vi "Untitled 11 (SubVI).vi"(6 "Number of SPI Buses in":i32, 7 "Device Info":T1, 8 "error in (no error)":errorcluster, 9 "VI to which to Add Engines and IO Nodes":path, 10 "LabVIEW Project to Script":path, 11 "Curent Bus Path":path) -> (0 "error out":errorcluster, 3 "Number of SPI Buses out":i32)   [LabVIEW 2014, in "SPI Engine Scripting.lvlib"]
uses:
  SPI Engine Scripting.lvlib
  State Machine/Controls/Device Information.ctl
  State Machine/Controls/Pin Information.ctl
  State Machine/Controls/Bus Information.ctl
  <vilib>/LabVIEW Icon API/API_Text.ctl
  <vilib>/LabVIEW Icon API/LabVIEW Icon API.lvlib
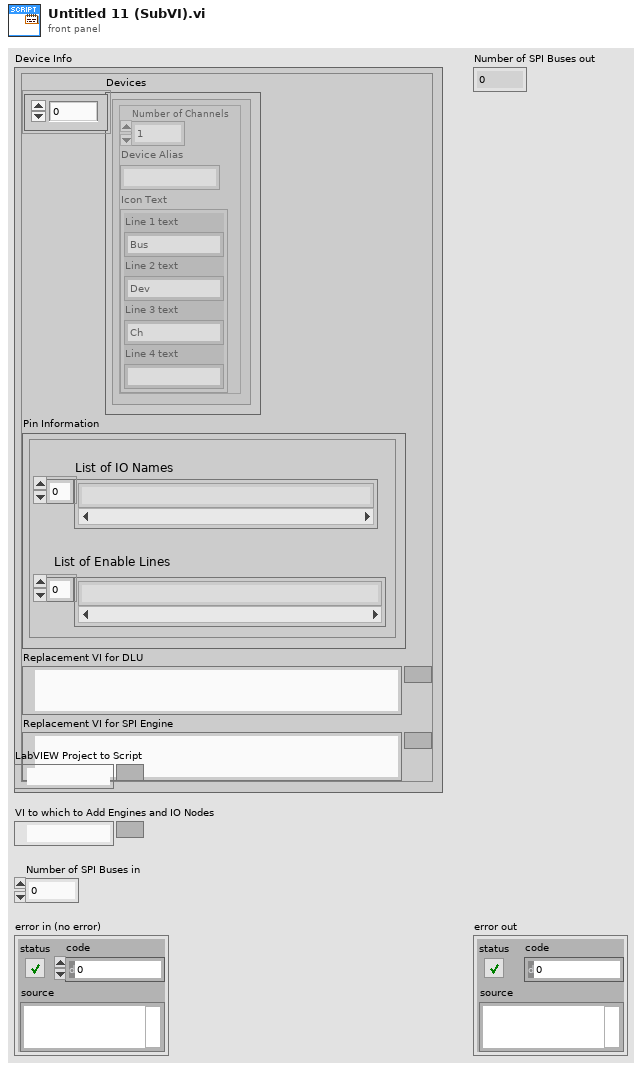
[diagram p1: front panel]
types:
  T1 = typedef "SPI Engine Scripting.lvlib/Bus Information.ctl" = cluster{"Devices":T2[], "Pin Information":T4, "Replacement VI for DLU":path, "Replacement VI for SPI Engine":path}
  T2 = typedef "Device Information.ctl" = cluster{"Number of Channels":i32, "Device Alias":string, "Icon Text":T3}
  T3 = typedef "LabVIEW Icon API.lvlib/API_Text.ctl" = cluster{"Line 1 text":string, "Line 2 text":string, "Line 3 text":string, "Line 4 text":string}
  T4 = typedef "Pin Information.ctl" = cluster{"List of IO Names":string[], "List of Enable Lines":string[]}
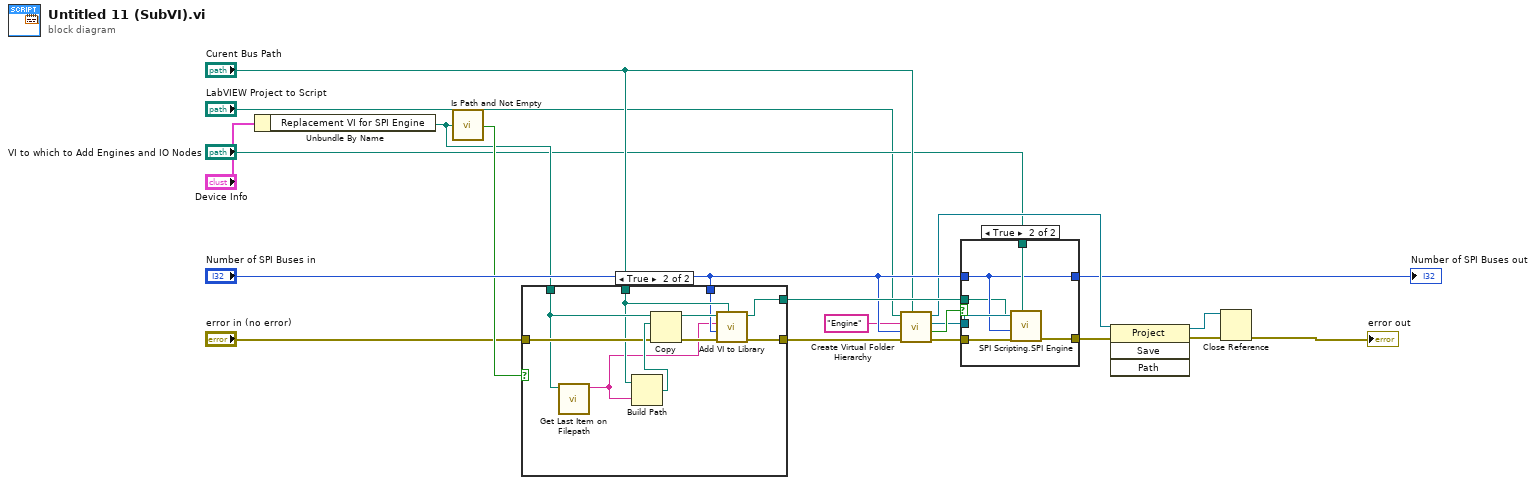
[diagram p0: block diagram]
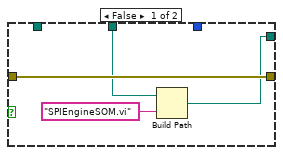
[diagram p2: hidden frame]
diagram:
  n1 = Unbundle By Name("Device Info") -> ("Replacement VI for SPI Engine"=w16:path)
  n2 = call <vilib>:"Is Path and Not Empty.vi"("path"=w16) -> ("Is Path and Not Empty?"=w18:bool)  [unwired: 4 in]
  n3 = case shown="True" w18 {
    tunnel: "error in (no error)" -> [w24 w31]
    tunnel: [w24 w30] -> w15
    tunnel: w16 -> [_ w29]
    tunnel: "Curent Bus Path" -> [w22 w28]
    tunnel: "Number of SPI Buses in" -> [_ w27]
    tunnel: [w21 w25] -> w20
    frame False {
      n4 = Build Path(base path=w22, name or relative path="SPIEngineSOM.vi" ("VI to Code Relative Path")) -> (appended path=w21:path)
    }
    frame True {
      n5 = call "Get Last Item on Filepath.vi"("Replacement VI for SPI Engine"=w29) -> ("String"=w26:string)  [unwired: 10 in]
      n6 = Build Path(base path=w28, name or relative path=w26) -> (appended path=w32:path)
      n7 = Copy(8:w31, 10:w32, 11:w29) -> (0:w34:errorcluster, 3:w33:path)  [unwired: 2 in, 1 out]
      n8 = call "Add VI to Library.vi"("Current Bus Path"=w28, "error in"=w34, "Bus Number"=w27, "VI Name"=w26, "Path to new VI"=w33) -> ("error out"=w30:errorcluster, "Path to new IO Node"=w25:path)  [unwired: 5 in]
    }
  }
  n9 = call "Create Virtual Folder Hierarchy.vi"(7:"Curent Bus Path", "error in"=w15, "Bus Number"="Number of SPI Buses in", "Virtual Folder Name"="Engine", "Path to Project"="LabVIEW Project to Script") -> ("error out"=w10:errorcluster, "FPGA Target Found"=w8:bool, "New Virtual Folder"=w7:refnum<vi>, "Project:Open"=w11:refnum<vi>)  [unwired: 3 in]
  n10 = case shown="True" w8 {
    tunnel: "VI to which to Add Engines and IO Nodes" -> [_ w42]
    tunnel: w10 -> [w36 w41]
    tunnel: "Number of SPI Buses in" -> [w35 w38]
    tunnel: [w36 w40] -> w9
    tunnel: w7 -> [_ w39]
    tunnel: [w35 w38] -> w4
    tunnel: w20 -> [_ w37]
    frame False {
    }
    frame True {
      n11 = call "SPI Scripting.SPI Engine.vi"("Path to Place SPI Engine"=w42, "error in"=w41, "Bus Number"=w38, 10:w39, "Path to Engine"=w37) -> ("error out"=w40:errorcluster)  [unwired: 6 in]
    }
  }
  "Number of SPI Buses out" <- w4
  n12 = invoke class="Project" method="Save"(reference=w11, error in=w9) -> (reference out=w13:refnum<vi>, error out=w12:errorcluster)  [unwired: 2 in, 2 out]
  n13 = Close Reference(reference=w13, error in (no error)=w12) -> (error out=→"error out":errorcluster)
